vi "Set PMT Power.vi"(8 "error in (no error)":errorcluster, 10 "Power Status":u32(ring), 11 "Handle":u32) -> (0 "error out":errorcluster, 3 "Status":i32)   [LabVIEW 2014, in "Photon Counter.lvlib" / "C8855-01.lvlib"]
doc: "Controls the power supply for the photon counting module connected to this unit.\n\n\n\n\nBOOL C8855API __stdcall C8855SetPmtPower(HANDLE hC8855,\n BYTE PowerStatus );"
uses:
  C8855-01.lvlib
  C8855-01api.dll
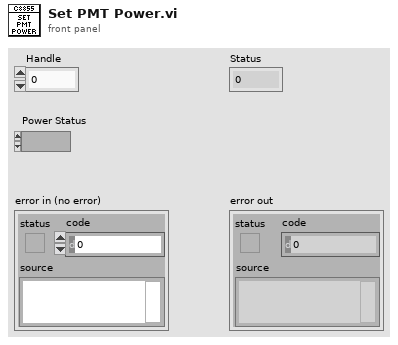
[diagram p1: front panel]
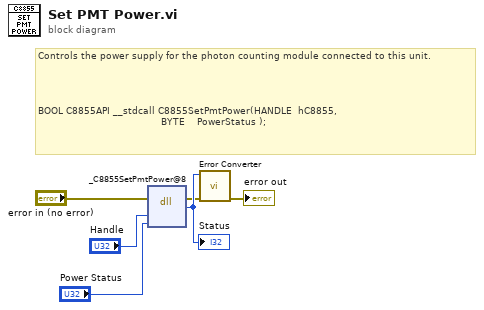
[diagram p0: block diagram]
diagram:
  # "Controls the power supply for the photon counting module connected to this unit.\n\n\n\n\nBOOL C8855API __stdcall C8855SetPmtPower(HANDLE\t hC8855,\n                                         BYTE    PowerStatus );"
  n1 = dll-call lib="C:/Users/Andy/Desktop/Trace Grabber/Drivers/C8855-01/C8855-01api.*" fn="_C8855SetPmtPower@8"(error in="error in (no error)", "Handle"="Handle", "Power Status"="Power Status") -> (error out=w2:errorcluster, w6:i32)  [unwired: 4 in, 1 out]
  "Status" <- w6
  n2 = call "Error Converter.vi"("error in (no error)"=w2, "error code"=w6) -> ("error out"=→"error out":errorcluster)  [unwired: 9 in]
